vi "Send Error API.vi"(8 "Error Cluster":errorcluster, 11 "Error":string) -> (0 "Error Out":errorcluster)   [LabVIEW 2017, in "Main controller.lvlib"]
uses:
  Main controller.lvlib
  Events/Controls/Error Data [cluster].ctl
  Events/Events.lvlib
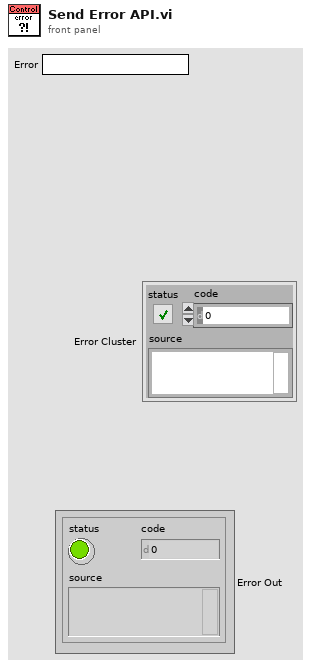
[diagram p1: front panel]
types:
  T1 = typedef "Events.lvlib/Error Data [cluster].ctl" = cluster{"Error":string, "Error Cluster":errorcluster}
  T2 = typedef "Events.lvlib/Refs [cluster].ctl" = cluster{"Exit":refnum<user-event>, "Controller":refnum<user-event>, "System Error":refnum<user-event>, "UI":refnum<user-event>, "Example Module":refnum<user-event>, "Shutter":refnum<user-event>, "Monochromator":refnum<user-event>, "DAQ":refnum<user-event>, "Scope":refnum<user-event>, "Processing":refnum<user-event>, "File IO":refnum<user-event>, "Colour wheel":refnum<user-event>}
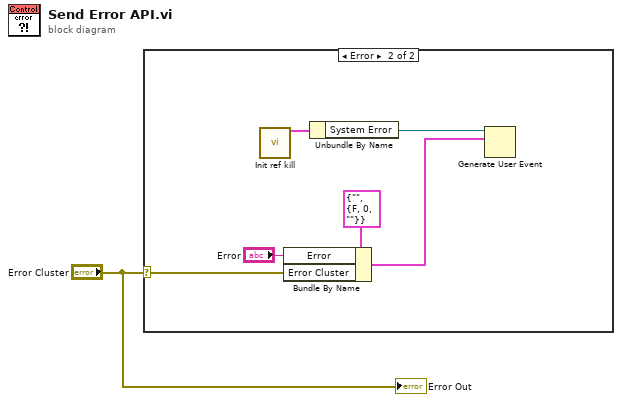
[diagram p0: block diagram]
diagram:
  n1 = case shown="Error" "Error Cluster" {
    selector: "Error Cluster" -> [_ w2]
    frame No Error {
    }
    frame Error {
      n2 = call "Init ref kill.vi"() -> ("Messages"=w7:T2)  [unwired: 10 in, 1 out]
      n3 = Bundle By Name(cluster=T1 {"Error"="", "Error Cluster"={"status"=FALSE, "code"=0, "source"=""}} ("event data"), "Error"="Error", "Error Cluster"=w2) -> (w4:T1)
      n4 = Unbundle By Name(w7) -> ("System Error"=w6:refnum<user-event>)
      n5 = Generate User Event(user event=w6, event data cluster=w4) -> ()  [unwired: 2 in, 2 out]
    }
  }
  "Error Out" <- "Error Cluster"
